vi "Dropper.vi"() -> ()   [LabVIEW 2016]
uses:
  <vilib>/DAQmx/write.llb/DAQmx Write (Analog 1D DBL 1Chan NSamp).vi
  <vilib>/DAQmx/create/channels.llb/DAQmx Create Channel (AO-Voltage-Basic).vi
  <vilib>/DAQmx/configure/timing.llb/DAQmx Timing (Sample Clock).vi
  <vilib>/DAQmx/miscellaneous.llb/DAQmx Fill In Error Info.vi
  <vilib>/Analysis/NI_AALBase.lvlib
panel:
  out "number of samples written per channel":u32
  out "Waveform Graph":dbl[](graph)
  out "error":i32
  in  "samples":i32=128
  in  "f1":dbl format="%0.2f"
  in  "f2":dbl=0.5 format="%0.2f"
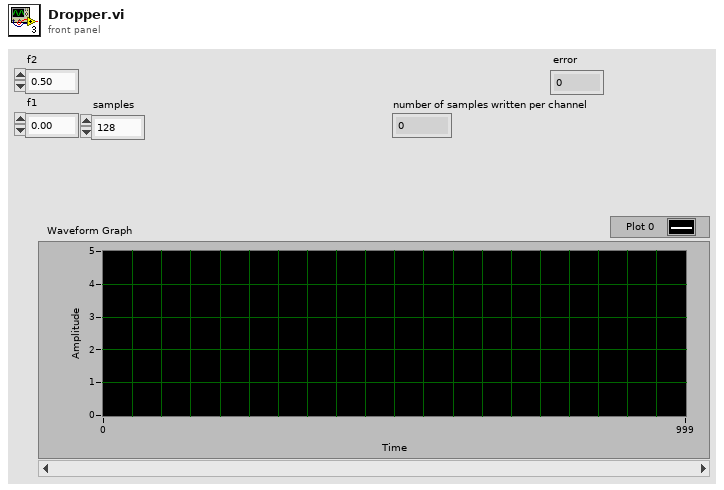
[diagram p1: front panel]
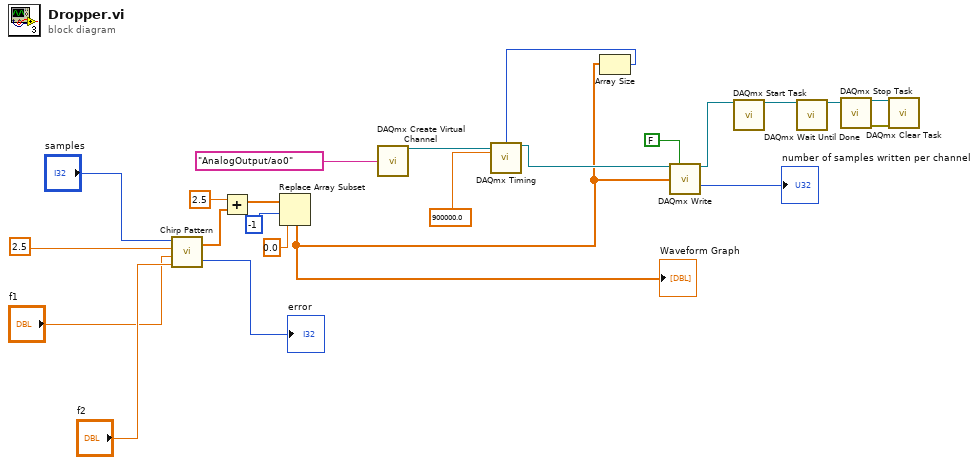
[diagram p0: block diagram]
diagram:
  n1 = call <vilib>:"Chirp Pattern.vi"("f2"="f2", "f1"="f1", "amplitude"=2.5, "samples"="samples") -> ("error"=→"error":i32, "Chirp Pattern"=w12:dbl[])
  n2 = Add(x=2.5, y=w12) -> (x+y=w11:dbl[])
  n3 = Replace Array Subset(array=w11, new element=0.0 ("new element/subarray"), index=-1) -> (w2:dbl[])
  "Waveform Graph" <- w2
  n4 = call-poly <vilib>:"DAQmx Create Virtual Channel.vi"("physical channels"=tag "AnalogOutput/ao0") -> ("task out"=w17:refnum<k21>)  [unwired: 13 in, 1 out]
  n5 = Array Size(array=w2) -> (size(s)=w1:i32)
  n6 = call-poly <vilib>:"DAQmx Timing.vi"("task/channels in"=w17, "samples per channel"=w1, "rate"=900000.0) -> ("task out"=w16:refnum<k21>)  [unwired: 11 in, 1 out]
  n7 = call-poly <vilib>:"DAQmx Write.vi"("task/channels in"=w16, "auto start"=FALSE, "data"=w2) -> ("task out"=w7:refnum<k21>, "number of samples written per channel"=→"number of samples written per channel":u32)  [unwired: 10 in, 1 out]
  n8 = call <vilib>:"DAQmx Start Task.vi"("task/channels in"=w7) -> ("task out"=w6:refnum<k21>)  [unwired: 13 in, 1 out]
  n9 = call <vilib>:"DAQmx Wait Until Done.vi"("task/channels in"=w6) -> ("task out"=w5:refnum<k21>)  [unwired: 13 in, 1 out]
  n10 = call <vilib>:"DAQmx Stop Task.vi"("task/channels in"=w5) -> ("task out"=w4:refnum<k21>, "error out"=w3:errorcluster)  [unwired: 13 in]
  n11 = call <vilib>:"DAQmx Clear Task.vi"("task in"=w4, "error in"=w3) -> ()  [unwired: 13 in, 1 out]
